vi "Method 2.vi"(8 "error in (no error)":errorcluster, 10 "My Input":dbl, 11 "Test Interface in":refnum<class "Test Async Interface.lvclass">) -> (0 "error out":errorcluster, 2 "My Output":dbl, 3 "Test Interface out":refnum<class "Test Async Interface.lvclass">)   [LabVIEW 2023, in "Test Async Interface.lvlib" / "Test Async Interface.lvclass"]
doc: "My Method Description"
uses:
  Test Async Interface.lvclass
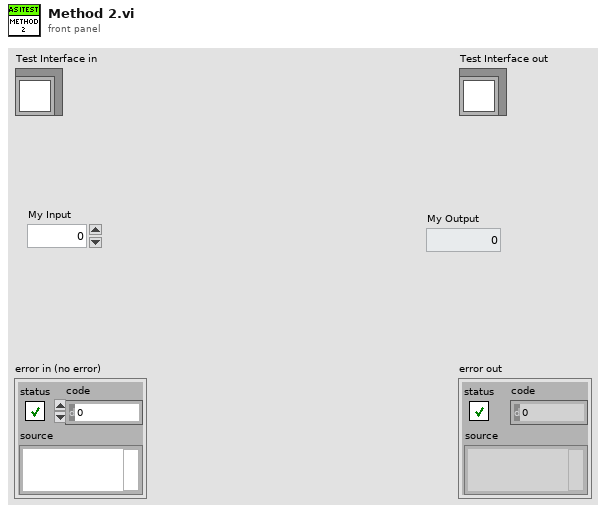
[diagram p1: front panel]
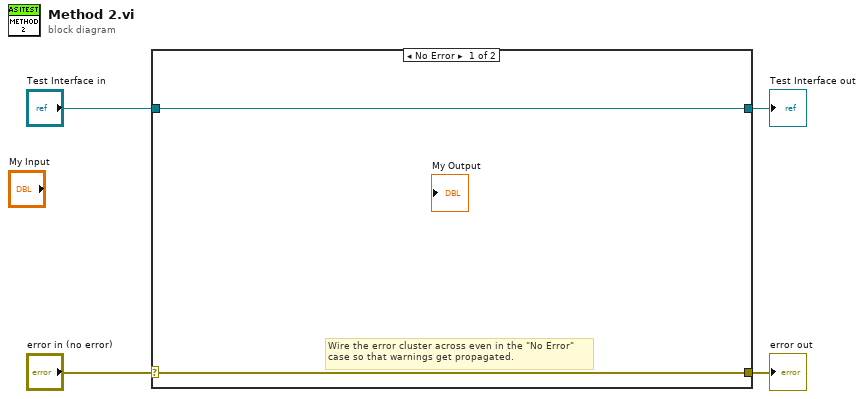
[diagram p0: block diagram]
diagram:
  n1 = case shown="No Error" "error in (no error)" {
    selector: "error in (no error)" -> [w5 w8]
    tunnel: [w5 w8] -> w3
    tunnel: [w6 w7] -> w1
    tunnel: "Test Interface in" -> [w6 w7]
    frame No Error {
      # "Wire the error cluster across even in the \"No Error\"\ncase so that warnings get propagated."
    }
    frame Error {
    }
  }
  "error out" <- w3
  "Test Interface out" <- w1
